vi "main_train.vi"() -> ()   [LabVIEW 2023]
panel:
  out "right":i32
  out "left":i32
  out "Numeric 3":i32
  out "Numeric 2":i32
  out "x-y*floor(x/y)":i32
  out "x = y?":bool
  out "return value":i32
  in  "stop":bool
  in  "start":bool
  out "error out":errorcluster
  in  "Pause Game":bool
  in  "Decrease\nPlayer Length":bool
  in  "Stop":bool
  out "p2 score":i32
  out "p1 score":i32
  in  "w_bool":bool
  in  "Down_bool":bool
  in  "s_bool":bool
  in  "Up_bool":bool
  out "game window":picture
  # "Player 1: W, S\nPlayer 2: Up, Down"
  # "Modifiers"
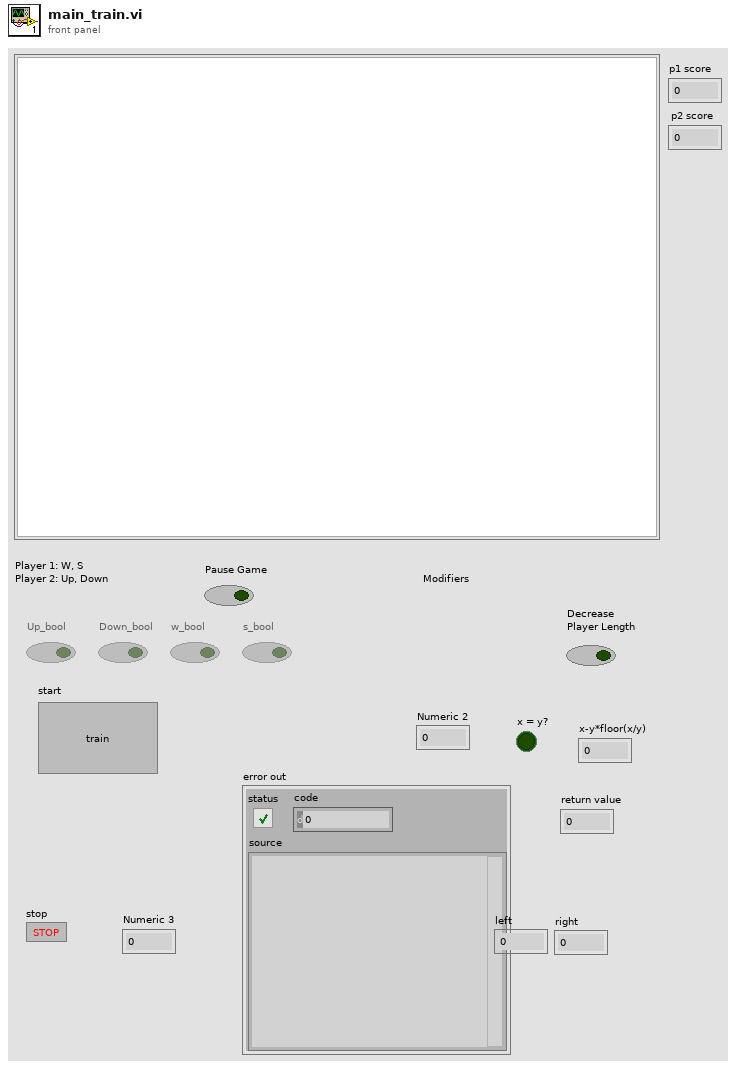
[diagram p1: front panel]
types:
  T1 = cluster{"output vector x":dbl, "output vector y":dbl}
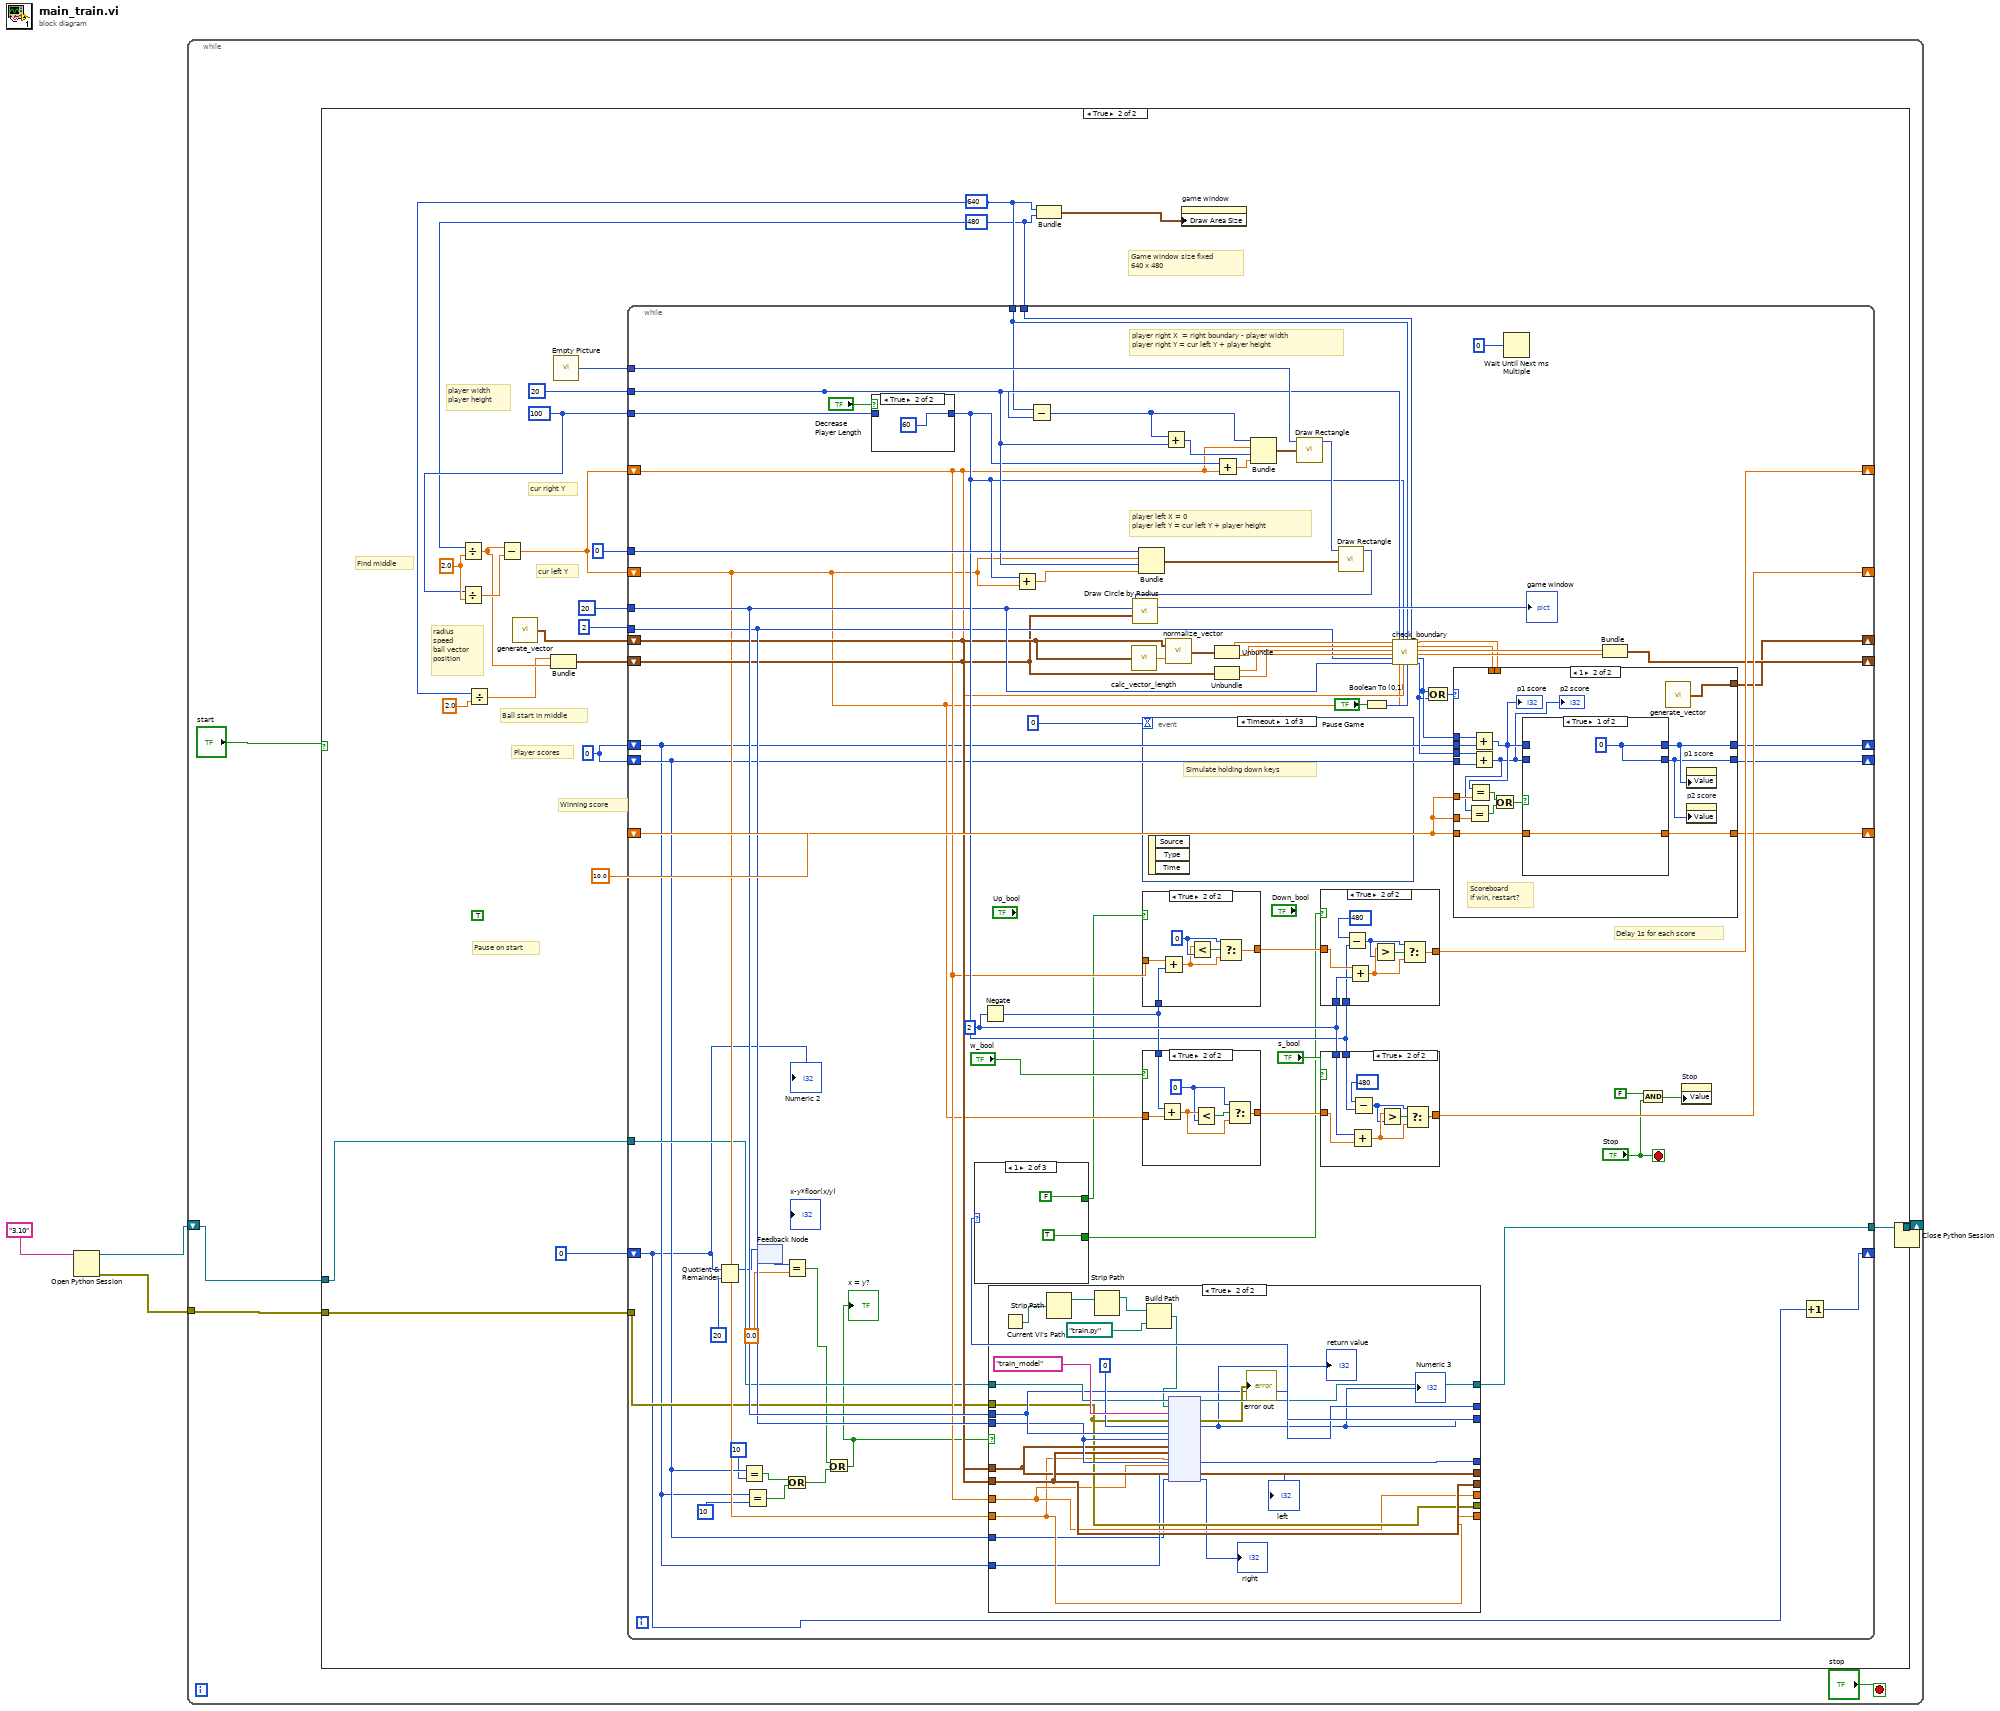
[diagram p0: block diagram]
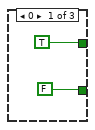
[diagram p3: hidden frame]
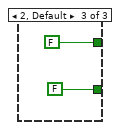
[diagram p4: hidden frame]
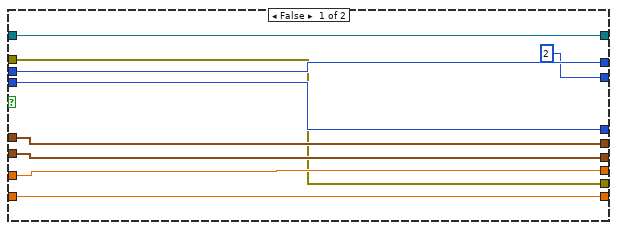
[diagram p5: hidden frame]
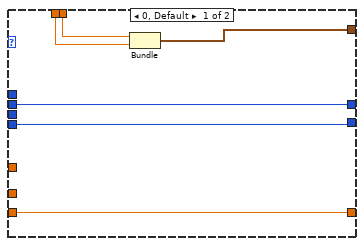
[diagram p7: hidden frame]
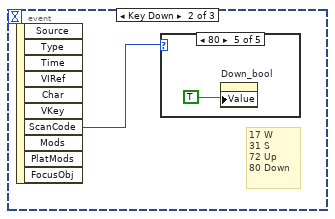
[diagram p13: hidden frame]
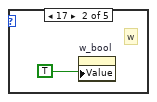
[diagram p15: hidden frame]
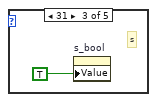
[diagram p16: hidden frame]
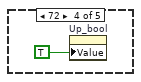
[diagram p17: hidden frame]
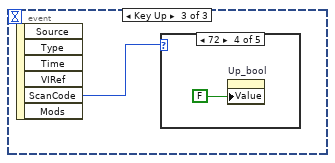
[diagram p18: hidden frame]
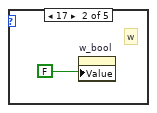
[diagram p20: hidden frame]
diagram:
  n1 = Open Python Session(python version="3.10" ("Python version")) -> (session out=w3:refnum<k35>, error out=w2:errorcluster)  [unwired: 2 in]
  n2 = while {
    tunnel: w2 -> [w7]
    shift-right: [w9] -> w4
    shift-left: w3 -> [w8]
    stop <- "stop" stop-if-true
    n3 = case shown="True" "start" {
      tunnel: [w10 w15] -> w9
      tunnel: w8 -> [w10 w12]
      tunnel: w7 -> [_ w13]
      frame False {
      }
      frame True {
        (unwired) TRUE ("Pause Game")
        w17 = 0
        w18 = 480
        w25 = 640
        w28 = 2.0 ("y")
        w26 = 100
        # "Pause on start"
        # "Winning score"
        # "Player scores"
        # "Ball start in middle"
        # "radius\nspeed\nball vector\nposition"
        # "Find middle"
        # "player width\nplayer height"
        # "cur left Y"
        # "cur right Y"
        # "Game window size fixed\n640 x 480"
        n4 = Divide(x=w18, y=w28) -> (x/y=w22:dbl)
        n5 = Divide(x=w26, y=w28) -> (x/y=w27:dbl)
        n6 = Divide(x=w25, y=2.0) -> (x/y=w21:dbl)
        n7 = Subtract(x=w22, y=w27) -> (x-y=w29:dbl)
        n8 = call "generate_vector.vi"() -> ("Cluster"=w16:cluster{"number":dbl, "number":dbl})
        n9 = Bundle(w21, w22) -> (w23:cluster{dbl, dbl})  [unwired: 1 in]
        n10 = call "Empty Picture"() -> ("empty picture"=w32:picture)
        n11 = while {
          tunnel: w25 -> [w83]
          tunnel: w32 -> [w108]
          shift-right: [w97] -> _
          shift-left: w29 -> [w55]
          shift-right: [w95] -> _
          shift-left: w29 -> [w54]
          tunnel: w26 -> [w65]
          tunnel: 20 -> [w84]
          tunnel: 0 -> [w106]
          shift-right: [w73] -> _
          shift-left: w16 -> [w57]
          shift-right: [w79] -> _
          shift-left: w23 -> [w56]
          tunnel: 20 -> [w60]
          tunnel: 2 -> [w59]
          tunnel: w18 -> [w82]
          shift-right: [w78] -> _
          shift-left: w17 -> [w43]
          shift-right: [w77] -> _
          shift-left: w17 -> [w45]
          shift-right: [w76] -> _
          shift-left: 10.0 ("upper limit") -> [w69]
          tunnel: [w58] -> w15
          tunnel: w13 -> [w53]
          tunnel: w12 -> [w52]
          shift-right: [w49] -> _
          shift-left: 0 -> [w34]
          stop <- "Stop" stop-if-true
          w100 = 2 ("y")
          # "Delay 1s for each score"
          # "player right X  = right boundary - player width\nplayer right Y = cur left Y + player height"
          # "player left X = 0\nplayer left Y = cur left Y + player height"
          n12 = Quotient & Remainder(x=w34, y=20) -> (x-y*floor(x/y)=w37:i32)  [unwired: 1 out]
          n13 = Equal?(x=w45, y=10) -> (x = y?=w40:bool)
          n14 = Equal?(x=w43, y=10) -> (x = y?=w41:bool)
          n15 = feedback-in #1(w37) -> ()
          n16 = feedback #1() -> (w36:i32)  [unwired: 1 in]
          n17 = Equal?(x=w36, y=0.0) -> (x = y?=w46:bool)
          n18 = Or(x=w40, y=w41) -> (x .or. y?=w39:bool)
          n19 = Or(x=w46, y=w39) -> (x .or. y?=w38:bool)
          "x = y?" <- w38
          n20 = case shown="True" "Decrease\nPlayer Length" {
            tunnel: w65 -> [w149 _]
            tunnel: [w149 60] -> w64
            frame False {
            }
            frame True {
            }
          }
          n21 = Negate(x=w100) -> (-x=w99:i32)
          n22 = case shown="True" w38 {
            tunnel: w60 -> [w125 w143]
            tunnel: w59 -> [w124 w142]
            tunnel: [w126 w147] -> w58
            tunnel: w57 -> [w123 w140]
            tunnel: w56 -> [w122 w141]
            tunnel: w55 -> [w121 w137]
            tunnel: w54 -> [w119 w136]
            tunnel: w53 -> [w120 w139]
            tunnel: w52 -> [w126 w145]
            tunnel: [w125 w143] -> _
            tunnel: [w124 w142] -> _
            tunnel: [w123 w140] -> _
            tunnel: [w122 w141] -> _
            tunnel: [w121 w137] -> _
            tunnel: [w120 w139] -> _
            tunnel: [w119 w136] -> _
            tunnel: [2 w138] -> w48
            tunnel: w45 -> [_ w134]
            tunnel: w43 -> [_ w135]
            frame False {
            }
            frame True {
              n23 = Current VI's Path() -> (path=w131:path)
              n24 = Strip Path(path=w131) -> (stripped path=w130:path)  [unwired: 1 out]
              n25 = Strip Path(path=w130) -> (stripped path=w129:path)  [unwired: 1 out]
              n26 = Build Path(base path=w129, name or relative path=path "train.py") -> (appended path=w127:path)
              n27 = node(w145, w127, "train_model" ("function name"), w139, 0, w143, w142, w140, w141, w136, w137, w135, w134) -> (w147:refnum<k35>, →"error out":errorcluster, w138:i32, →"left":i32, →"right":i32)  [unwired: 6 in, 2 out]
              "return value" <- w138
              "Numeric 3" <- w138
            }
          }
          n28 = case shown="1" w48 {
            tunnel: [TRUE FALSE FALSE] -> w35
            tunnel: [FALSE TRUE FALSE] -> w47
            frame 0 {
            }
            frame 1 {
            }
            frame 2, Default {
            }
          }
          n29 = Add(x=w64, y=w54) -> (x+y=w105:dbl)
          n30 = Subtract(x=w83, y=w84) -> (x-y=w111:i32)
          n31 = call "calc_vector_length.vi"("vector"=w57) -> ("length"=w89:dbl)
          n32 = Bundle(w106, w54, w84, w105) -> (w104:cluster{i32, dbl, i32, dbl})  [unwired: 1 in]
          n33 = event shown="[0] Timeout" {
            selector: _ -> [_ _ _]
            dyn-events: _ -> [_ _ _]
            timeout: 0 -> [_ _ _]
            event Timeout {
              # "Simulate holding down keys"
              n34 = event-data() -> ()  [unwired: 1 in, 3 out]
            }
            event Key Down {
              # "17 W\n31 S\n72 Up\n80 Down"
              n35 = event-data() -> ("ScanCode"=w210:i16)  [unwired: 1 in, 9 out]
              n36 = case shown="80" w210 {
                frame 0, Default {
                }
                frame 17 {
                  # "w"
                  n37 = property on="w_bool" class="Bool (strict)"("Value"=TRUE) -> ()  [unwired: 2 in, 2 out]
                }
                frame 31 {
                  # "s"
                  n38 = property on="s_bool" class="Bool (strict)"("Value"=TRUE) -> ()  [unwired: 2 in, 2 out]
                }
                frame 72 {
                  n39 = property on="Up_bool" class="Bool (strict)"("Value"=TRUE) -> ()  [unwired: 2 in, 2 out]
                }
                frame 80 {
                  n40 = property on="Down_bool" class="Bool (strict)"("Value"=TRUE) -> ()  [unwired: 2 in, 2 out]
                }
              }
            }
            event Key Up {
              n41 = event-data() -> ("ScanCode"=w215:i16)  [unwired: 1 in, 5 out]
              n42 = case shown="72" w215 {
                frame 0, Default {
                }
                frame 17 {
                  # "w"
                  n43 = property on="w_bool" class="Bool (strict)"("Value"=FALSE) -> ()  [unwired: 2 in, 2 out]
                }
                frame 31 {
                  # "s"
                  n44 = property on="s_bool" class="Bool (strict)"("Value"=FALSE) -> ()  [unwired: 2 in, 2 out]
                }
                frame 72 {
                  n45 = property on="Up_bool" class="Bool (strict)"("Value"=FALSE) -> ()  [unwired: 2 in, 2 out]
                }
                frame 80 {
                  n46 = property on="Down_bool" class="Bool (strict)"("Value"=FALSE) -> ()  [unwired: 2 in, 2 out]
                }
              }
            }
          }
          n47 = case shown="True" w35 {
            tunnel: w99 -> [_ w205]
            tunnel: w55 -> [w203 w206]
            tunnel: [w203 w204] -> w98
            frame False {
            }
            frame True {
              w208 = 0 ("y")
              n48 = Add(x=w206, y=w205) -> (x+y=w207:dbl)
              n49 = Less?(x=w207, y=w208) -> (x < y?=w209:bool)
              n50 = Select(t=w208, s=w209, f=w207) -> (s? t:f=w204:dbl)
            }
          }
          n51 = case shown="True" "w_bool" {
            tunnel: w54 -> [w196 w198]
            tunnel: w99 -> [_ w199]
            tunnel: [w196 w197] -> w96
            frame False {
            }
            frame True {
              w200 = 0 ("y")
              n52 = Add(x=w199, y=w198) -> (x+y=w202:dbl)
              n53 = Less?(x=w202, y=w200) -> (x < y?=w201:bool)
              n54 = Select(t=w200, s=w201, f=w202) -> (s? t:f=w197:dbl)
            }
          }
          n55 = Add(x=w111, y=w84) -> (x+y=w110:i32)
          n56 = call "normalize_vector.vi"("Numeric"=w89, "vector"=w57) -> ("output"=w90:cluster{"x":dbl, "y":dbl})
          n57 = Unbundle(w90) -> ("x"=w88:dbl, "y"=w87:dbl)
          n58 = Unbundle(w56) -> (w86:dbl, w85:dbl)
          n59 = Add(x=w64, y=w55) -> (x+y=w109:dbl)
          n60 = Bundle(w111, w55, w110, w109) -> (w107:cluster{i32, dbl, i32, dbl})  [unwired: 1 in]
          n61 = call <vilib>:"Draw Rectangle.vi"("picture"=w108, "rect"=w107) -> ("new picture"=w103:picture)  [unwired: 7 in]
          n62 = case shown="True" w47 {
            tunnel: w100 -> [_ w191]
            tunnel: w98 -> [w187 w190]
            tunnel: [w187 w189] -> w97
            tunnel: w64 -> [_ w188]
            frame False {
            }
            frame True {
              n63 = Subtract(x=480 ("y"), y=w188) -> (x-y=w193:i32)
              n64 = Add(x=w190, y=w191) -> (x+y=w194:dbl)
              n65 = Greater?(x=w194, y=w193) -> (0:w195:bool)
              n66 = Select(t=w193, s=w195, f=w194) -> (s? t:f=w189:dbl)
            }
          }
          n67 = case shown="True" "s_bool" {
            tunnel: w100 -> [_ w181]
            tunnel: w96 -> [w178 w182]
            tunnel: [w178 w180] -> w95
            tunnel: w64 -> [_ w179]
            frame False {
            }
            frame True {
              n68 = Add(x=w181, y=w182) -> (x+y=w185:dbl)
              n69 = Subtract(x=480 ("y"), y=w179) -> (x-y=w184:i32)
              n70 = Greater?(x=w185, y=w184) -> (0:w186:bool)
              n71 = Select(t=w184, s=w186, f=w185) -> (s? t:f=w180:dbl)
            }
          }
          n72 = call <vilib>:"Draw Rectangle.vi"("picture"=w103, "rect"=w104) -> ("new picture"=w92:picture)  [unwired: 7 in]
          n73 = call <vilib>:"Draw Circle by Radius.vi"("pixel center"=w56, "radius"=w60, "picture"=w92) -> ("new picture"=→"game window":picture)  [unwired: 8 in]
          n74 = Boolean To (0,1)(Boolean="Pause Game") -> (0, 1=w61:i16)
          n75 = call "check_boundary.vi"("vector x"=w88, "vector y"=w87, "position x"=w86, "position y"=w85, "speed"=w59, "radius"=w60, "player width"=w84, "player left position y"=w54, "player height"=w64, "player right position y"=w55, "window width"=w83, "pause"=w61, "window height"=w82) -> ("output vector x"=w75:dbl, "output vector y"=w74:dbl, "output x"=w81:dbl, "output y"=w80:dbl, "left win"=w67:i32, "right win"=w66:i32)  [unwired: 1 in]
          n76 = Compound Arithmetic op=OR(w67, w66) -> (w68:i32)
          n77 = case shown="1" w68 {
            tunnel: w43 -> [w156 w163]
            tunnel: w45 -> [w155 w161]
            tunnel: w67 -> [_ w164]
            tunnel: w66 -> [_ w162]
            tunnel: [w156 w158] -> w78
            tunnel: [w155 w157] -> w77
            tunnel: w69 -> [_ w172]
            tunnel: w69 -> [_ w171]
            tunnel: [w154 w167] -> w76
            tunnel: w69 -> [w154 w166]
            tunnel: w75 -> [w153 _]
            tunnel: w74 -> [w152 _]
            tunnel: [w151 w165] -> w73
            frame 0, Default {
              n78 = Bundle("output vector x"=w153, "output vector y"=w152) -> (w151:T1)  [unwired: 1 in]
            }
            frame 1 {
              # "Scoreboard\nIf win, restart?"
              n79 = Add(x=w164, y=w163) -> (x+y=w160:i32)
              "p1 score" <- w160
              n80 = Equal?(x=w160, y=w172) -> (x = y?=w169:bool)
              n81 = Add(x=w162, y=w161) -> (x+y=w159:i32)
              "p2 score" <- w159
              n82 = Equal?(x=w159, y=w171) -> (x = y?=w168:bool)
              n83 = Or(x=w169, y=w168) -> (x .or. y?=w170:bool)
              n84 = case shown="True" w170 {
                tunnel: [w174 w175] -> w157
                tunnel: [w174 w176] -> w158
                tunnel: [w173 w177] -> w167
                tunnel: w166 -> [w173 w177]
                tunnel: w160 -> [_ w176]
                tunnel: w159 -> [_ w175]
                frame True {
                  w174 = 0
                }
                frame False {
                }
              }
              n85 = call "generate_vector.vi"() -> ("Cluster"=w165:cluster{"number":dbl, "number":dbl})
              n86 = property on="p1 score" class="DigNum (strict)"("Value"=w158) -> ()  [unwired: 2 in, 2 out]
              n87 = property on="p2 score" class="DigNum (strict)"("Value"=w157) -> ()  [unwired: 2 in, 2 out]
            }
          }
          n88 = Wait Until Next ms Multiple(millisecond multiple=u32 0 ("milliseconds to wait")) -> ()  [unwired: 1 out]
          n89 = Bundle("output x"=w81, "output y"=w80) -> (w79:cluster{"output x":dbl, "output y":dbl})  [unwired: 1 in]
          n90 = And(x=FALSE, y="Stop") -> (x .and. y?=w70:bool)
          n91 = property on="Stop" class="Bool (strict)"("Value"=w70) -> ()  [unwired: 2 in, 2 out]
          n92 = Increment(x=w34) -> (x+1=w49:i32)
          "Numeric 2" <- w34
        }
        n93 = Bundle(w25, w18) -> (w33:cluster{i32, i32})  [unwired: 1 in]
        n94 = property on="game window" class="Pict"("Draw Area Size"=w33) -> ()  [unwired: 2 in, 2 out]
      }
    }
  }
  n95 = Close Python Session(session in=w4) -> ()  [unwired: 1 in, 1 out]
